vi "AssignControlToTerminal.vi"(3 "error in (no error)":errorcluster, 4 "connPaneIndex":i32, 5 "dup targetVI in":refnum<vi>, 6 "Control in":refnum<vi>) -> (0 "error out":errorcluster, 1 "Control out":refnum<vi>, 2 "VI out":refnum<vi>)   [LabVIEW 2013]
uses:
  <vilib>/Utility/miscctls.llb/LVPositionTypeDef.ctl
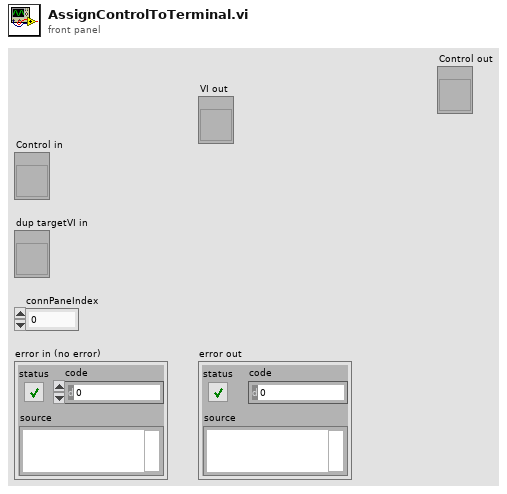
[diagram p1: front panel]
types:
  T1 = typedef "LVPositionTypeDef.ctl" = cluster{"Left":i32, "Top":i32}
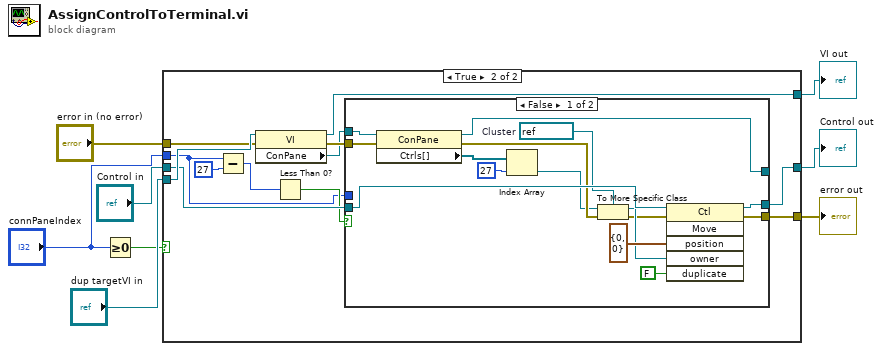
[diagram p0: block diagram]
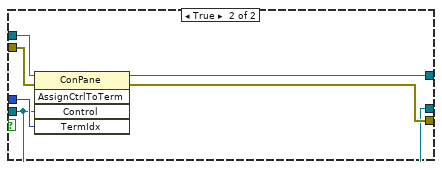
[diagram p3: hidden frame]
diagram:
  n1 = Greater Or Equal To 0?(x="connPaneIndex") -> (x >= 0?=w3:bool)
  n2 = case shown="True" w3 {
    tunnel: "dup targetVI in" -> [w11 w23]
    tunnel: "error in (no error)" -> [w10 w22]
    tunnel: [w11 w21] -> w6
    tunnel: "connPaneIndex" -> [_ w14]
    tunnel: [w10 w13] -> w7
    tunnel: "Control in" -> [w9 w18]
    tunnel: [w9 w12] -> w1
    frame False {
    }
    frame True {
      n3 = Subtract(x=w14, y=27) -> (x-y=w15:i32)
      n4 = property class="VI"(reference=w23, error in=w22) -> (reference out=w21:refnum<vi>, error out=w20:errorcluster, "ConPane"=w19:refnum<vi>)
      n5 = Less Than 0?(x=w15) -> (x < 0?=w17:bool)
      n6 = case shown="False" w17 {
        tunnel: w20 -> [w36 w44]
        tunnel: [w25 w43] -> w13
        tunnel: [w32 w42] -> _
        tunnel: w19 -> [w35 w41]
        tunnel: w18 -> [w38 w39]
        tunnel: w14 -> [_ w40]
        tunnel: [w24 w39] -> w12
        frame False {
          w28 = refnum<vi> refnum  # Cluster
          n7 = property class="ConPane"(reference=w35, error in=w36) -> (reference out=w32:refnum<vi>, error out=w30:errorcluster, "Ctrls[]"=w34:refnum<vi>[])
          n8 = Index Array(array=w34, index=27) -> (element=w29:refnum<vi>)
          n9 = To More Specific Class(target class=w28, reference=w29, error in=w30) -> (specific class reference=w27:refnum<vi>, error out=w26:errorcluster)
          n10 = invoke class="Ctl" method="Move"(reference=w38, error in=w26, "position"=T1 {"Left"=0, "Top"=0}, "owner"=w27, "duplicate"=FALSE ("Duplicate? (F)")) -> (reference out=w24:refnum<vi>, error out=w25:errorcluster)  [unwired: 1 in, 4 out]
        }
        frame True {
          n11 = invoke class="ConPane" method="AssignCtrlToTerm"(reference=w41, error in=w44, "Control"=w39, "TermIdx"=w40) -> (reference out=w42:refnum<vi>, error out=w43:errorcluster)  [unwired: 1 in, 3 out]
        }
      }
    }
  }
  "error out" <- w7
  "VI out" <- w6
  "Control out" <- w1
